vi "Module Init.vi"(8 "error in (no error)":errorcluster, 11 "Log Manager Module in":refnum<class "Log Manager Module.lvclass">) -> (0 "error out":errorcluster, 3 "Log Manager Module out":refnum<class "Log Manager Module.lvclass">)   [LabVIEW 2020, in "VolatusData.lvlib" / "Log Manager Module.lvclass"]
uses:
  Log Manager Module.lvclass
  C:/dev/lv20CE/relink/lv-volatus/Volatus/Module/Module.lvclass
  Volatus/Message Registration.ctl
  Volatus/Module/Module.lvclass/Module.ctl
  VolatusConfig/VolatusConfigElement/VolatusConfigElement.lvclass/VolatusConfigElement.ctl
  Log Manager Module.lvclass/Log Manager Module.ctl
  Volatus/Module/Config.vi
  VolatusConfig/VolatusConfigElement/Element.vi
  VolatusConfig/Task/Task Config.lvclass
  C:/dev/lv20CE/relink/lv-volatus/VolatusConfig/VolatusConfigElement/VolatusConfigElement.lvclass
  VolatusConfig/VolatusConfigElement/VolatusConfigElement.lvclass
  lv-cdm/CDM-Config/Config Element/Config Element.lvclass
  Volatus/Volatus.lvlib
  Volatus/Module/Module.lvclass
  C:/dev/lv20CE/relink/lv-volatus/VolatusData/Log Manager Module/Log Manager Module.lvclass
  lv-vecto/Vecto/Group DBL/Group DBL.lvclass
  C:/dev/lv20CE/relink/lv-volatus/VolatusConfig/Task/Task Config.lvclass
  C:/dev/lv20CE/relink/lv-vecto/Vecto/Group/Group.lvclass
  C:/dev/lv20CE/relink/lv-vecto/Vecto/Group DBL/Group DBL.lvclass
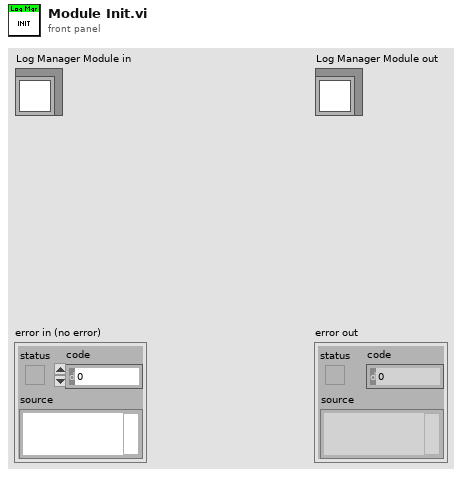
[diagram p1: front panel]
types:
  T1 = typedef "Volatus.lvlib/Message Registration.ctl" = cluster{"Message Type":string, "Message ID":string}
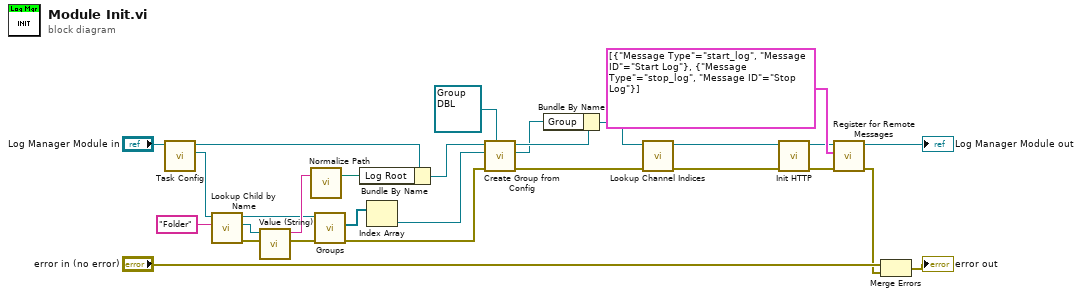
[diagram p0: block diagram]
diagram:
  n1 = call "Task Config.vi"("Module in"="Log Manager Module in") -> ("Task Config"=w26:refnum<class "Task Config.lvclass">, "Module out"=w27:refnum<class "Log Manager Module.lvclass">)  [unwired: 8 in, 1 out]
  n2 = call "Lookup Child by Name.vi"("Child Name"="Folder", "VolatusConfigElement in"=w26) -> ("error out"=w24:errorcluster, "Child"=w23:refnum<class "Config Element.lvclass">, "VolatusConfigElement out"=w14:refnum<class "Task Config.lvclass">)  [unwired: 6 in, 1 out]
  n3 = call "Value (String).vi"("error in (no error)"=w24, "Config Element in"=w23) -> ("error out"=w15:errorcluster, "String Value"=w22:string)  [unwired: 8 in]
  n4 = call "Normalize Path.vi"("Path String"=w22) -> ("Path"=w21:path)  [unwired: 2 in]
  n5 = call "Groups.vi"("error in (no error)"=w15, "Task in"=w14) -> ("error out"=w9:errorcluster, "Groups"=w13:refnum<class "Group Config.lvclass">[])  [unwired: 7 in, 1 out]
  n6 = Bundle By Name(cluster=w27, "Log Root"=w21) -> (w11:refnum<class "Log Manager Module.lvclass">)
  n7 = Index Array(array=w13) -> (element=w12:refnum<class "Group Config.lvclass">)  [unwired: 1 in]
  n8 = call "Create Group from Config.vi"("Group Type (Abstract)"=refnum<class "Group DBL.lvclass"> refnum ("Vecto.lvlib:StringGroup.lvclass"), "error in (no error)"=w9, "Group Config"=w12, "Module in"=w11) -> ("error out"=w8:errorcluster, "Group"=w6:refnum<class "Group DBL.lvclass">, "Module out"=w10:refnum<class "Log Manager Module.lvclass">)  [unwired: 5 in]
  n9 = Bundle By Name(cluster=w10, "Group"=w6) -> (w4:refnum<class "Log Manager Module.lvclass">)
  n10 = call "Lookup Channel Indices.vi"("error in (no error)"=w8, "Log Manager Module in"=w4) -> ("error out"=w5:errorcluster, "Log Manager Module out"=w2:refnum<class "Log Manager Module.lvclass">)  [unwired: 8 in]
  n11 = call "Init HTTP.vi"("error in (no error)"=w5, "Log Manager Module in"=w2) -> ("error out"=w3:errorcluster, "Log Manager Module out"=w1:refnum<class "Log Manager Module.lvclass">)  [unwired: 8 in]
  n12 = call "Register for Remote Messages.vi"("error in (no error)"=w3, "Messages"=T1[] [{"Message Type"="start_log", "Message ID"="Start Log"}, {"Message Type"="stop_log", "Message ID"="Stop Log"}], "Module in"=w1) -> ("error out"=w16:errorcluster, "Module out"=→"Log Manager Module out":refnum<class "Log Manager Module.lvclass">)  [unwired: 7 in]
  n13 = Merge Errors("error in (no error)", w16) -> (→"error out":errorcluster)
